vi "LCS kNN1.vi"() -> ()   [LabVIEW 2014]
panel:
  out "LCS/min (Lsample,Lknown)":dbl[][](array[numeric])
  out "Distance values (LCS)":dbl[][](array[numeric])
  in  "All data in 2":string[][](array[string])=array2046x3[6138 elements]
  out "size(s)":i32
  out "accuracy":string[][](array[string])
  out "Results":string[][](array[string])
  out "Training data (K)":string[][](array[string])
  out "test data K-1":string[][](array[string])
  in  "K folds K":i32=10
  out "K folds data":string[][](array[string])
  out "Assigned using LCS (enhanced)":string[][](array[string])
  out "Assigned using LCS":string[][](array[string])
  in  "class labels for training data":string[](array[string])
  in  "kNN k":i32=5
  in  "training data (cluster centers)":string[](array[string])
  in  "test data (patterns in)":string[](array[string])=["0 4 0", "4 0 4", "0 4 0", "4 0 4", "0 4 0", "4 0 4", "0 4 0", "4 0 -2", "0 -2 3", "-2 3 0", "3 0 3", "0 3 0", "3 0 4", "0 4 0", "-2 0 1", "0 1 0", "1 0 -4", "0 -4 4", "-2 2 0", "2 0 -1", "0 -1 -4", "-1 -4 1", "-4 1 0", "1 0 3", "0 3 0", "-1 0 -1", "0 -1 2", "0 -1 1", "-1 1 0", "1 0 4", "0 4 0", "4 0 3", "0 3 -2", "3 -2 0", "-2 0 -2", "0 -2 3", "-2 3 -2", "3 -2 0", "-2 0 4", "0 4 0", "4 0 -2", "0 -2 2", "2 -1 0", "-1 0 4", "0 4 0", "4 0 2", "0 2 0", "2 0 -2", "0 -2 0", "1 -1 0", "-1 0 3", "0 3 0", "3 0 -4", "0 -4 4", "-4 4 -4", "4 -4 0", "2 -1 0", "-1 0 3", "0 3 -2", "3 -2 0", "-2 0 -3", "0 -3 0", "-3 0 3", "0 3 0", "3 0 -3", "0 -3 0", "0 4 0", "4 0 4", "0 4 -4", "4 -4 1", "-4 1 -1", "1 -1 0", "-1 0 -3", "0 -3 0", "-3 0 1", "0 1 -4", "1 -4 1", "-4 1 0", "1 0 4", "0 4 0", "4 0 -4", "0 -4 0", "-4 0 -4", "0 -4 4", "-4 4 -4", "4 -4 1", "0 -4 1", "-4 1 0", "1 0 -4", "0 -4 4", "0 4 0", "4 0 -2", "0 -2 2", "-2 2 -2", "2 -2 2", "-2 2 -2", "2 -2 2", "-2 2 -1", "2 -1 0", "-1 0 4", "0 4 0", "4 0 2", "0 2 0", "2 0 4", "0 4 0", "4 0 2", "0 2 -2", "2 -2 0", "-2 0 4", "1 0 -1", "0 -1 0", "-1 0 -1", "0 -1 0", "-1 0 1", "0 1 -1", "-2 2 -2", "2 -2 3", "1 0 -1", "0 -1 0", "-1 0 -1", "0 -1 2", "-1 2 0", "2 0 2", "0 2 -2", "2 -2 0", "-2 0 -4", "0 -4 0", "-2 2 0", "2 0 3", "0 3 -2", "3 -2 2", "1 -1 0", "-1 0 3", "0 4 0", "-2 0 1", "0 1 -4", "1 -4 0", "-4 0 -3", "0 -3 0", "1 0 -1", "0 -1 2", "-1 2 -1", "2 -1 1", "-1 1 -4", "-2 0 -1", "0 -1 1", "0 3 0", "3 0 3", "0 3 0", "3 0 3", "0 3 -2", "-4 0 -4", "0 -4 4", "0 4 0", "4 0 -4", "0 -4 0", "-4 0 -4", "-2 2 0", "2 0 4", "0 4 -4", "4 -4 0", "-4 0 2", "0 2 -2"]
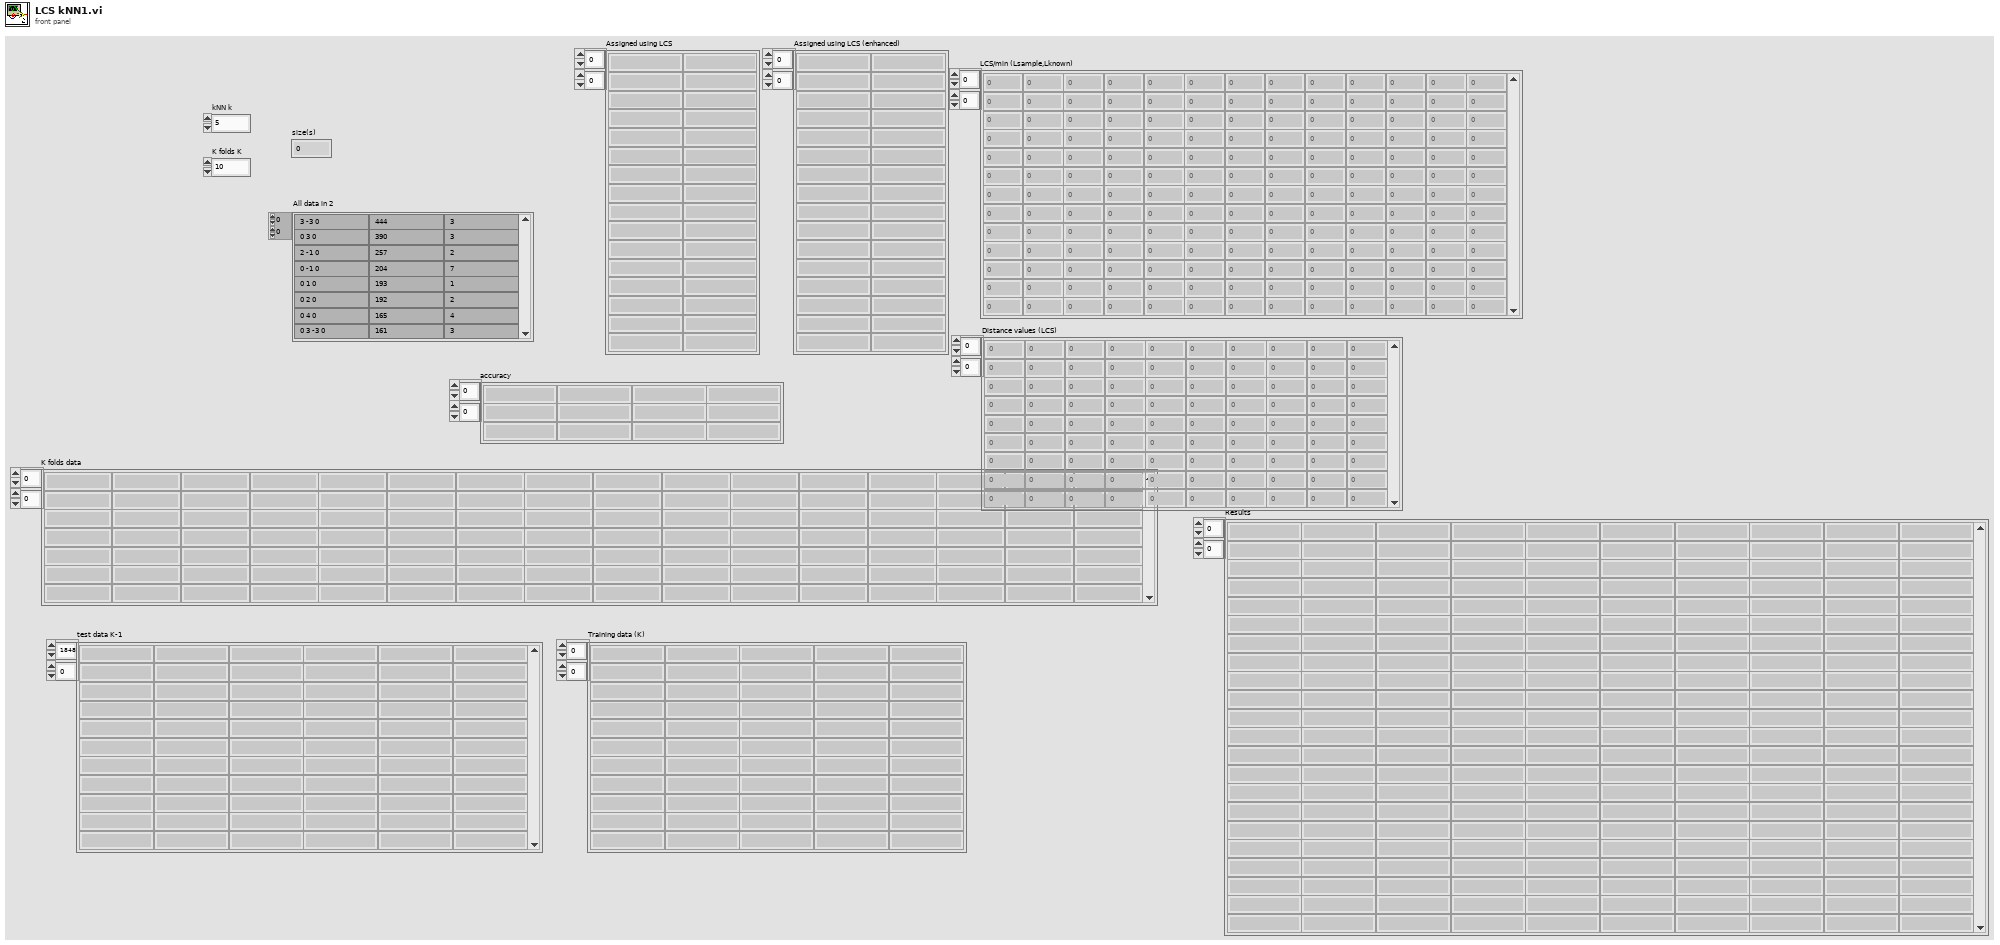
[diagram p1: front panel]
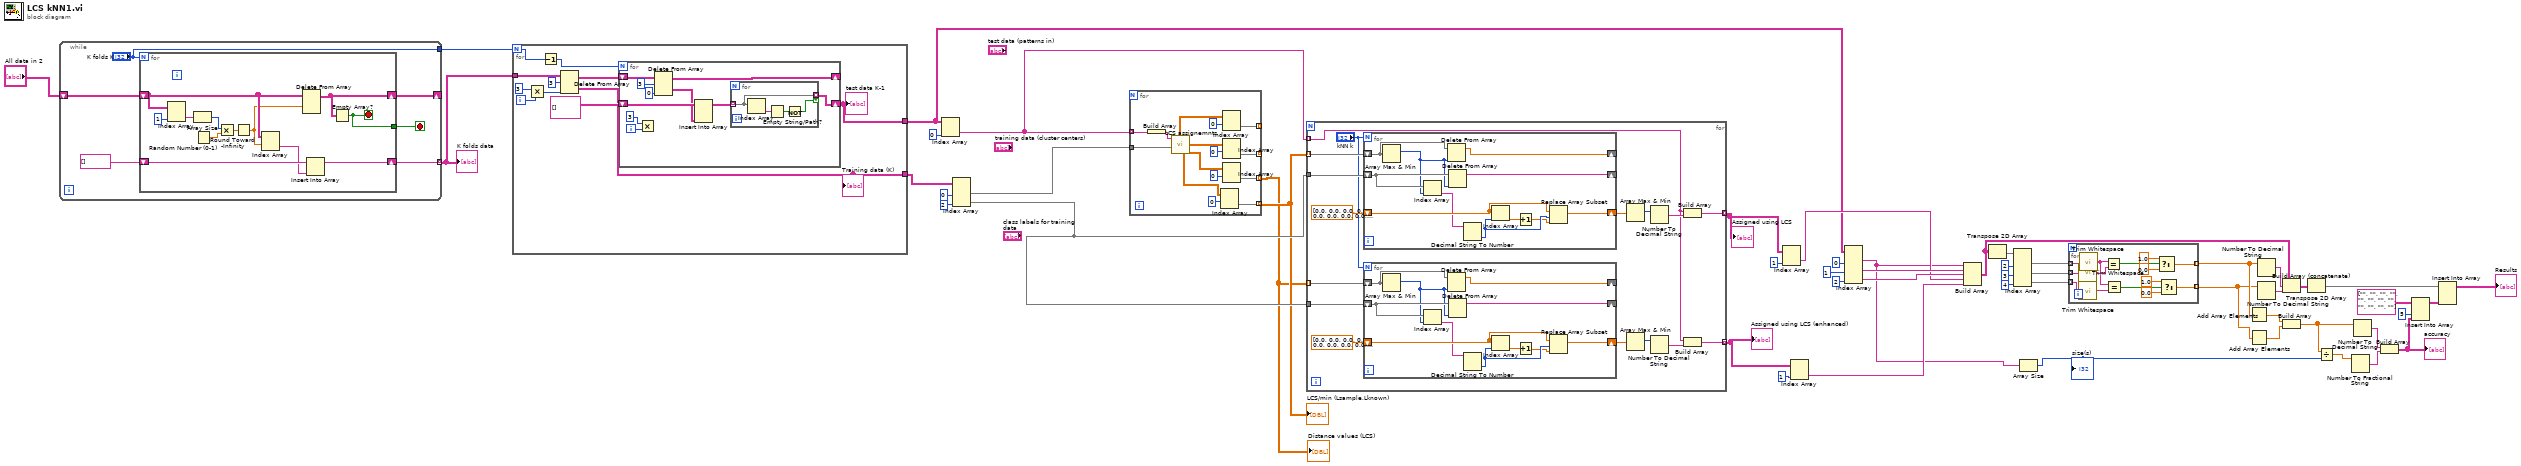
[diagram p0: block diagram]
diagram:
  n1 = while {
    shift-right: [w54] -> _
    shift-left: "All data in 2" -> [w55]
    tunnel: [w56] -> w51 mode=indexing
    tunnel: ["K folds K"] -> w50
    stop <- w53 stop-if-true
    n2 = for {
      N: "K folds K" -> [_]
      shift-right: [w62] -> w56
      shift-left: string[] [] ("all rows 2") -> [w69]
      shift-right: [w60] -> w54
      shift-left: w55 -> [w61]
      tunnel: [w59] -> w53
      stop <- w59 stop-if-true
      n3 = Index Array(array=w61, index (col)=1 ("disabled index (col)")) -> (element=w65:string[])  [unwired: 1 in]
      n4 = Array Size(array=w65) -> (size(s)=w66:i32)
      n5 = Random Number (0-1)() -> (number: 0 to 1=w67:dbl)
      n6 = Multiply(x=w66, y=w67) -> (x*y=w68:dbl)
      n7 = Round Toward -Infinity(1:w68) -> (0:w58:dbl)
      n8 = Index Array(array=w61, index (row)=w58) -> (element=w63:string[])  [unwired: 1 in]
      n9 = Delete From Array(array=w61, index (row)=w58) -> (array with subset deleted=w60:string[][])  [unwired: 2 in, 1 out]
      n10 = Insert Into Array(array=w69, new element=w63) -> (w62:string[])  [unwired: 1 in]
      n11 = Empty Array?(array=w60) -> (empty?=w59:bool)
    }
  }
  "K folds data" <- w51
  n12 = for {
    N: w50 -> [w73]
    tunnel: w51 -> [w80]
    tunnel: [w71] -> w11
    tunnel: [w70] -> w7
    i -> [w78]
    n13 = Multiply(x=3, y=w78) -> (x*y=w76:i32)
    n14 = Decrement(x=w73) -> (x-1=w72:i32)
    n15 = Delete From Array(array=w80, length=3, index (col)=w76) -> (deleted portion=w71:string[][], array with subset deleted=w75:string[][])  [unwired: 1 in]
    "Training data (K)" <- w71
    n16 = for {
      N: w72 -> [_]
      shift-right: [w81] -> w70
      shift-left: string[][] [] ("all rows 2") -> [w89]
      shift-right: [w84] -> _
      shift-left: w75 -> [w90]
      i -> [w86]
      n17 = Multiply(x=3, y=w86) -> ()  [unwired: 1 out]
      n18 = Delete From Array(array=w90, length=3 ("index (col)"), index (col)=0 ("disabled index (col)")) -> (deleted portion=w88:string[][], array with subset deleted=w84:string[][])  [unwired: 1 in]
      n19 = Insert Into Array(array=w89, new element=w88) -> (w82:string[][])  [unwired: 2 in]
      n20 = for {
        tunnel: w82 -> [w93] mode=indexing
        tunnel: [w93] -> w81 mode=indexing if=w94
        n21 = Index Array(array=w93) -> (element=w92:string)  [unwired: 1 in]
        n22 = Empty String/Path?(string/path=w92) -> (empty?=w91:bool)
        n23 = Not(x=w91) -> (.not. x?=w94:bool)
      }
    }
    "test data K-1" <- w70
  }
  n24 = Index Array(array=w7, index (col)=0 ("disabled index (col)")) -> (element=w13:string[])  [unwired: 1 in]
  n25 = Index Array(array=w11, index (col) #1=0 ("disabled index (col)"), index (col) #2=2 ("index (col)")) -> (element #1=w8:string[], element #2=w9:string[])  [unwired: 2 in]
  n26 = for {
    tunnel: w13 -> [w108] mode=indexing
    tunnel: w8 -> [w109]
    tunnel: [w104] -> _ mode=indexing
    tunnel: [w102] -> w1 mode=indexing
    tunnel: [w100] -> w2 mode=indexing
    tunnel: [w98] -> _ mode=indexing
    n27 = Build Array(w108) -> (w107:string[])
    n28 = call "LCS assignemnts.vi"("cluster centers"=w109, "Patterns in"=w107) -> ("LCS/Lsample (zeroed)/Lknown"=w95:dbl[][], "LCS/Lsample/Lknown"=w106:dbl[][], "Distance values (LCS)"=w96:dbl[][], "LCS/MAX (Lsample,Lknown) 2"=w97:dbl[][])  [unwired: 3 in, 3 out]
    n29 = Index Array(array=w96, index (row)=0) -> (element=w100:dbl[])  [unwired: 1 in]
    n30 = Index Array(array=w97, index (row)=0) -> (element=w98:dbl[])  [unwired: 1 in]
    n31 = Index Array(array=w106, index (row)=0) -> (element=w104:dbl[])  [unwired: 1 in]
    n32 = Index Array(array=w95, index (row)=0) -> (element=w102:dbl[])  [unwired: 1 in]
  }
  "Distance values (LCS)" <- w1
  "LCS/min (Lsample,Lknown)" <- w2
  n33 = for {
    tunnel: w13 -> [w115] mode=indexing
    tunnel: w2 -> [w125] mode=indexing
    tunnel: w9 -> [w124]
    tunnel: w1 -> [w114] mode=indexing
    tunnel: w9 -> [w113]
    tunnel: [w112] -> w20 mode=indexing
    tunnel: [w111] -> w16 mode=indexing
    n34 = for {
      N: "kNN k" -> [_]
      shift-right: [w144] -> _
      shift-left: w125 -> [w147]
      shift-right: [w143] -> _
      shift-left: w124 -> [w146]
      shift-right: [w138] -> w121
      shift-left: dbl[] [0.0, 0.0, 0.0, 0.0, 0.0, 0.0, 0.0, 0.0, 0.0, 0.0, 0.0, 0.0] -> [w139]
      n35 = Array Max & Min(array=w147) -> (max index (indices)=w145:i32)  [unwired: 3 out]
      n36 = Index Array(array=w146, index=w145) -> (element=w137:string)
      n37 = Delete From Array(array=w147, index=w145) -> (array with subset deleted=w144:dbl[])  [unwired: 1 in, 1 out]
      n38 = Delete From Array(array=w146, index=w145) -> (array with subset deleted=w143:string[])  [unwired: 1 in, 1 out]
      n39 = Decimal String To Number(string=w137) -> (number=w142:i32)  [unwired: 2 in, 1 out]
      n40 = Index Array(array=w139, index=w142) -> (element=w140:dbl)
      n41 = Increment(x=w140) -> (x+1=w141:dbl)
      n42 = Replace Array Subset(array=w139, new element=w141, index=w142) -> (w138:dbl[])
    }
    n43 = for {
      N: "kNN k" -> [_]
      shift-right: [w133] -> _
      shift-left: w114 -> [w136]
      shift-right: [w132] -> _
      shift-left: w113 -> [w135]
      shift-right: [w127] -> w118
      shift-left: dbl[] [0.0, 0.0, 0.0, 0.0, 0.0, 0.0, 0.0, 0.0, 0.0, 0.0, 0.0, 0.0] -> [w128]
      n44 = Array Max & Min(array=w136) -> (max index (indices)=w134:i32)  [unwired: 3 out]
      n45 = Index Array(array=w135, index=w134) -> (element=w126:string)
      n46 = Delete From Array(array=w136, index=w134) -> (array with subset deleted=w133:dbl[])  [unwired: 1 in, 1 out]
      n47 = Delete From Array(array=w135, index=w134) -> (array with subset deleted=w132:string[])  [unwired: 1 in, 1 out]
      n48 = Decimal String To Number(string=w126) -> (number=w131:i32)  [unwired: 2 in, 1 out]
      n49 = Index Array(array=w128, index=w131) -> (element=w129:dbl)
      n50 = Increment(x=w129) -> (x+1=w130:dbl)
      n51 = Replace Array Subset(array=w128, new element=w130, index=w131) -> (w127:dbl[])
    }
    n52 = Array Max & Min(array=w121) -> (max index (indices)=w122:i32)  [unwired: 3 out]
    n53 = Array Max & Min(array=w118) -> (max index (indices)=w117:i32)  [unwired: 3 out]
    n54 = Number To Decimal String(number=w122) -> (decimal integer string=w120:string)  [unwired: 1 in]
    n55 = Number To Decimal String(number=w117) -> (decimal integer string=w119:string)  [unwired: 1 in]
    n56 = Build Array(w115, w120) -> (w112:string[])
    n57 = Build Array(w115, w119) -> (w111:string[])
  }
  "Assigned using LCS" <- w20
  "Assigned using LCS (enhanced)" <- w16
  n58 = Index Array(array=w20, index (col)=1 ("disabled index (col)")) -> (element=w18:string[])  [unwired: 1 in]
  n59 = Index Array(array=w16, index (col)=1 ("disabled index (col)")) -> (element=w15:string[])  [unwired: 1 in]
  n60 = Index Array(array=w7, index (col) #1=0 ("disabled index (col)"), index (col) #2=1 ("index (col)"), index (col) #3=2 ("index (col)")) -> (element #1=w5:string[], element #2=w23:string[], element #3=w22:string[])  [unwired: 3 in]
  n61 = Build Array(w5, w23, w22, w18, w15) -> (w6:string[][])
  n62 = Transpose 2D Array(2D array=w6) -> (transposed array=w41:string[][])
  n63 = Index Array(array=w41, index (col) #1=2 ("disabled index (col)"), index (col) #2=3 ("index (col)"), index (col) #3=4 ("index (col)")) -> (element #1=w44:string[], element #2=w43:string[], element #3=w42:string[])  [unwired: 3 in]
  n64 = Array Size(array=w5) -> (size(s)=w4:i32)
  "size(s)" <- w4
  n65 = for {
    tunnel: w44 -> [w153] mode=indexing
    tunnel: w43 -> [w152] mode=indexing
    tunnel: w42 -> [w151] mode=indexing
    tunnel: [w155] -> w26 mode=indexing
    tunnel: [w154] -> w25 mode=indexing
    n66 = call <vilib>:"Trim Whitespace.vi"("string"=w152) -> ("trimmed string"=w150:string)  [unwired: 1 in]
    n67 = call <vilib>:"Trim Whitespace.vi"("string"=w151) -> ("trimmed string"=w149:string)  [unwired: 1 in]
    n68 = call <vilib>:"Trim Whitespace.vi"("string"=w153) -> ("trimmed string"=w148:string)  [unwired: 1 in]
    n69 = Equal?(x=w148, y=w150) -> (x = y?=w161:bool)
    n70 = Equal?(x=w148, y=w149) -> (x = y?=w156:bool)
    n71 = Select(t=1.0, s=w161, f=0.0) -> (s? t:f=w155:dbl)
    n72 = Select(t=1.0, s=w156, f=0.0) -> (s? t:f=w154:dbl)
  }
  n73 = Add Array Elements(numeric array=w26) -> (sum=w27:dbl)
  n74 = Add Array Elements(numeric array=w25) -> (sum=w28:dbl)
  n75 = Number To Decimal String(number=w26) -> (decimal integer string=w40:string[])  [unwired: 1 in]
  n76 = Number To Decimal String(number=w25) -> (decimal integer string=w39:string[])  [unwired: 1 in]
  n77 = Build Array (concatenate)(w6, w40, w39) -> (w38:string[][])
  n78 = Build Array(w27, w28) -> (w29:dbl[])
  n79 = Transpose 2D Array(2D array=w38) -> (transposed array=w24:string[][])
  n80 = Divide(x=w29, y=w4) -> (x/y=w30:dbl[])
  n81 = Number To Fractional String(number=w30) -> (F-format string=w32:string[])  [unwired: 3 in]
  n82 = Number To Decimal String(number=w29) -> (decimal integer string=w31:string[])  [unwired: 1 in]
  n83 = Build Array(w31, w32) -> (w36:string[][])
  "accuracy" <- w36
  n84 = Insert Into Array(array=string[][] [["", "", "", "", "", ""], ["", "", "", "", "", ""]] ("appended array 3"), index (col)=5 ("disabled index (col)"), new element=w36) -> (w35:string[][])  [unwired: 1 in]
  n85 = Insert Into Array(array=w24, new element=w35) -> (→"Results":string[][])  [unwired: 2 in]
